vi "Check Last Modified.vi"(6 "Last-Modified":timestamp, 8 "error in (no error)":errorcluster, 10 "Target Path":string, 11 "Caching in":refnum<class "Caching.lvclass">) -> (0 "error out":errorcluster, 1 "From Cache?":bool, 2 "Response":refnum<class "Response.lvclass">, 3 "Caching out":refnum<class "Caching.lvclass">)   [LabVIEW 2020, in "HTTP Server.lvlib" / "Caching.lvclass"]
uses:
  Caching.lvclass
  Caching.lvclass/Caching.ctl
  lv-http-util/HTTP Utils/Response/Response.lvclass
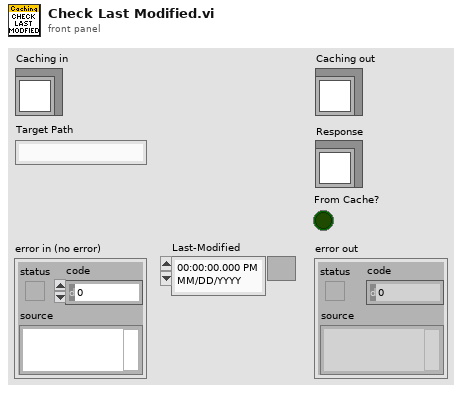
[diagram p1: front panel]
types:
  T1 = typedef "HTTP Server.lvlib/Caching.lvclass/Cache Item.ctl" = cluster{"ID":string, "File":bool, "Path":path, "Value":string, "Created":timestamp, "Expires":timestamp}
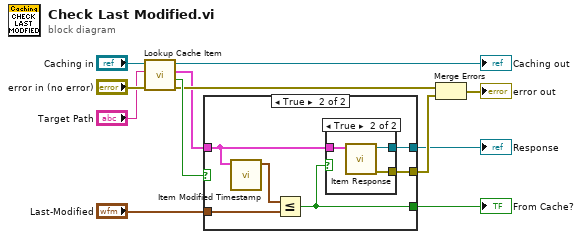
[diagram p0: block diagram]
diagram:
  n1 = call "Lookup Cache Item.vi"("error in (no error)"="error in (no error)", "ID"="Target Path", "Caching in"="Caching in") -> ("error out"=w11:errorcluster, "Found?"=w12:bool, "Cache Item"=w4:T1, "Caching out"=→"Caching out":refnum<class "Caching.lvclass">)  [unwired: 5 in]
  n2 = case shown="True" w12 {
    tunnel: w4 -> [_ w14]
    tunnel: "Last-Modified" -> [_ w18]
    tunnel: [_ w17] -> w1
    tunnel: [_ w16] -> w2
    tunnel: [_ w15] -> w10
    frame False {
    }
    frame True {
      n3 = call "Item Modified Timestamp.vi"("Cache Item"=w14) -> ("Modified"=w13:timestamp)  [unwired: 10 in]
      n4 = Less Or Equal?(x=w13, y=w18) -> (x <= y?=w17:bool)
      n5 = case shown="True" w17 {
        tunnel: w14 -> [_ w21]
        tunnel: [_ w20] -> w16
        tunnel: [_ w19] -> w15
        frame False {
        }
        frame True {
          n6 = call "Item Response.vi"("Cache Item"=w21) -> ("error out"=w19:errorcluster, "Response"=w20:refnum<class "Response.lvclass">)  [unwired: 9 in]
        }
      }
    }
  }
  "Response" <- w2
  "From Cache?" <- w1
  n7 = Merge Errors(w11, w10) -> (→"error out":errorcluster)
